vi "Configure Sequencer List Increment.vi"(7 "List Increment (Dwell Time)":i32(ring) items=["Dwell Time", "ARB Cycles", "User Action", "Measurement", "Trigger"], 8 "error in (no error)":errorcluster, 9 "Index (0)":i32, 10 "Instance (1)":i32=1, 11 "VISA resource name":refnum<visa-resource-name>) -> (0 "error out":errorcluster, 3 "VISA resource name out":refnum<visa-resource-name>)   [LabVIEW 2015, in "Rohde&Schwarz CMXP GPRF.lvlib"]
doc: "Defines the list increment for the sequencer list entry with the selected Index.\n\nAttribute:\nRSCMXPGPRF_ATTR_SEQUENCER_LIST_INCREMENT\n\nRemote-control command:\nSOURce:GPRF:GEN<i>:SEQuencer:LIST:LINCrement"
uses:
  <instrlib>/Rohde&Schwarz CMXP GPRF/Rohde&Schwarz CMXP GPRF.lvlib
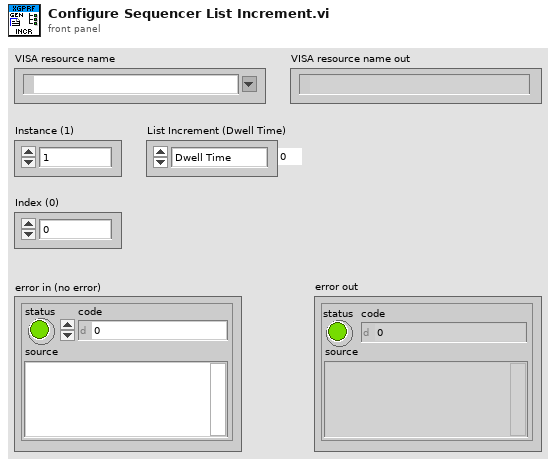
[diagram p1: front panel]
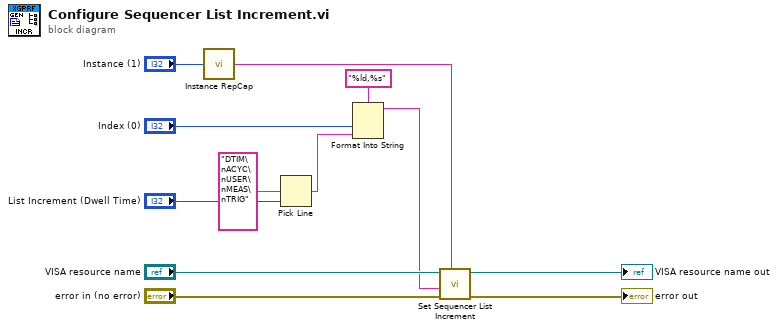
[diagram p0: block diagram]
diagram:
  n1 = call <instrlib>:"Instance RepCap.vi"("instance  in"="Instance (1)") -> ("instance out"=w11:string)
  n2 = Pick Line(multi-line string="DTIM\nACYC\nUSER\nMEAS\nTRIG" ("format string"), line index="List Increment (Dwell Time)") -> (output string=w2:string)  [unwired: 1 in]
  n3 = Format Into String(format string="%ld,%s", "Index (0)", w2) -> (resulting string=w1:string)  [unwired: 2 in, 1 out]
  n4 = call "Set Sequencer List Increment"("Repeated Capabilities"=w11, "error in (no error)"="error in (no error)", "Sequencer List Increment ()"=w1, "instrument handle"="VISA resource name") -> ("error out"=→"error out":errorcluster, "instrument handle out"=→"VISA resource name out":refnum<visa-resource-name>)  [unwired: 6 in]
